vi "IntakeGetDemands.vi"() -> (0 "turntableDemand":dbl, 1 "intakeLowerDemand":dbl, 2 "intakeUpperDemand":dbl, 3 "IntakeDown":bool)   [LabVIEW 2020]
doc: "Gets Intake global variables\n\nOutputs\n--intakeUpperDemand--Double\n--intakeUpperDemand--Double\n--turntableDemand--Double"
uses:
  IntakeGlobal.vi
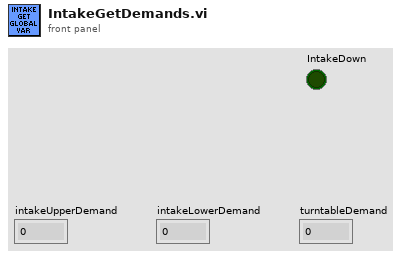
[diagram p1: front panel]
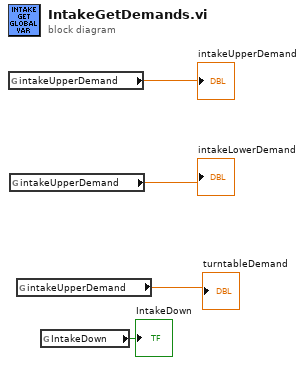
[diagram p0: block diagram]
diagram:
  n1 = global read "IntakeGlobal.vi" "intakeUpperDemand"() -> (→"intakeUpperDemand":dbl)
  n2 = global read "IntakeGlobal.vi" "intakeUpperDemand"() -> (→"intakeLowerDemand":dbl)
  n3 = global read "IntakeGlobal.vi" "intakeUpperDemand"() -> (→"turntableDemand":dbl)
  n4 = global read "IntakeGlobal.vi" "IntakeDown"() -> (→"IntakeDown":bool)
